vi "Launch PLC Handler.vi"(8 "error in (no error)":errorcluster, 11 "Controller in":refnum<class "Controller.lvclass">) -> (0 "error out":errorcluster, 3 "Controller out":refnum<class "Controller.lvclass">)   [LabVIEW 2022 SP3, in "Controller.lvlib" / "Controller.lvclass"]
uses:
  Controller.lvclass
  C:/Program Files/National Instruments/LabVIEW 2022/vi.lib/ActorFramework/Actor/Actor.lvclass
  PLCHandler/PLCHandler/PLCHandler.lvclass
  Controller.lvclass/Controller.ctl
  UserInterface/UserInterface Messages/Log Data Msg/Log Data Msg.lvclass/Log Data Msg.ctl
  <vilib>/ActorFramework/Message Enqueuer/Message Enqueuer.lvclass/Message Enqueuer.ctl
  <vilib>/ActorFramework/Message Enqueuer/Enqueue.vi
  UserInterface/UserInterface Messages/Log Data Msg/Log Data Msg.lvclass
  C:/Program Files/National Instruments/LabVIEW 2022/vi.lib/ActorFramework/Message/Message.lvclass
  PLCHandler/PLCHandler Messages/Init Msg/Init Msg.lvclass
  <vilib>/ActorFramework/Message Priority Queue/Priority Enqueue.vi
  <vilib>/ActorFramework/Actor/Actor.lvclass
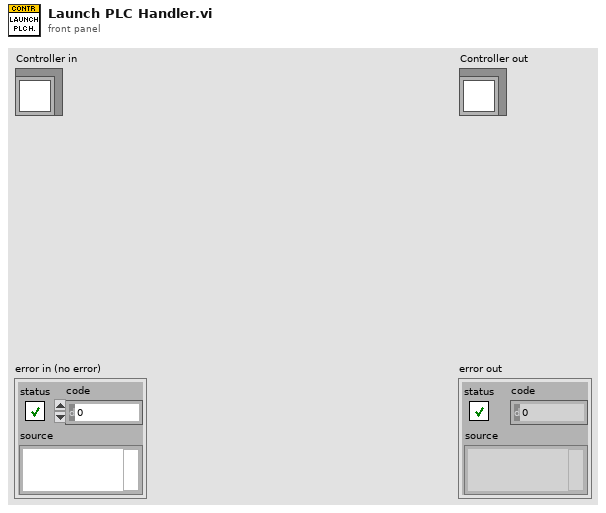
[diagram p1: front panel]
types:
  T1 = typedef "PLC Settings.ctl" = cluster{"Port":refnum<visa-resource-name>, "BaudRate":u32, "Wakeup Signal Address ":dbl, "Acquisiton Address":dbl, "Acknowledgement Address":dbl, "Sleep Address":dbl}
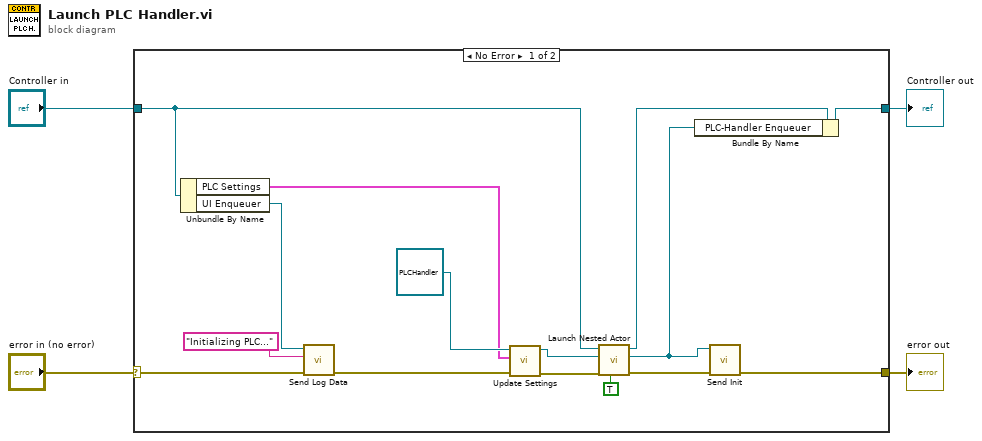
[diagram p0: block diagram]
diagram:
  n1 = case shown="No Error" "error in (no error)" {
    selector: "error in (no error)" -> [w7 w21]
    tunnel: [w10 w21] -> w3
    tunnel: [w18 w20] -> w1
    tunnel: "Controller in" -> [w17 w20]
    frame No Error {
      n2 = Unbundle By Name(w17) -> ("PLC Settings"=w13:T1, "UI Enqueuer"=w5:refnum<class "Message Enqueuer.lvclass">)
      n3 = call "Send Log Data.vi"("error in (no error)"=w7, "Message"="Initializing PLC...", "Message Enqueuer"=w5) -> ("error out"=w6:errorcluster)  [unwired: 7 in, 1 out]
      n4 = call "Update Settings.vi"("error in (no error)"=w6, "Settings"=w13, "PLCHandler in"=refnum<class "PLCHandler.lvclass"> refnum ("PLCHandler.lvlib:PLCHandler.lvclass")) -> ("error out"=w14:errorcluster, "PLCHandler out"=w15:refnum<class "PLCHandler.lvclass">)  [unwired: 7 in]
      n5 = call <vilib>:"Launch Nested Actor.vi"("Open Actor Core front panel? (F)"=TRUE, "error in (no error)"=w14, "Nested Actor"=w15, "Caller Actor in"=w17) -> ("error out"=w11:errorcluster, "Nested Actor's Enqueuer"=w12:refnum<class "Message Enqueuer.lvclass">, "Caller Actor out"=w9:refnum<class "Controller.lvclass">)  [unwired: 5 in]
      n6 = Bundle By Name(cluster=w9, "PLC-Handler Enqueuer"=w12) -> (w18:refnum<class "Controller.lvclass">)
      n7 = call "Send Init.vi"("error in (no error)"=w11, "Message Enqueuer"=w12) -> ("error out"=w10:errorcluster)  [unwired: 8 in, 1 out]
    }
    frame Error {
    }
  }
  "error out" <- w3
  "Controller out" <- w1
